vi "Echo.vi"(4 "Magnitude":dbl=0.5, 6 "Delay ms:":i32=5000, 7 "Input":path) -> (5 "output":path)   [LabVIEW 2012]
panel:
  out "Waveform Graph 2":waveform(dbl)(graph)
  out "Waveform Graph":waveform(dbl)(graph)
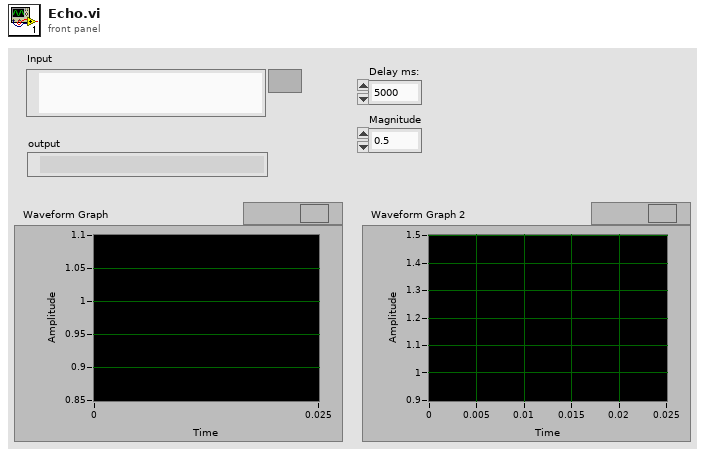
[diagram p1: front panel]
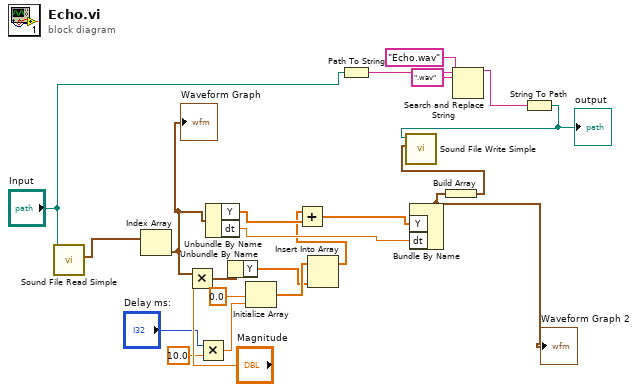
[diagram p0: block diagram]
diagram:
  n1 = call <vilib>:"Sound File Read Simple.vi"("path"="Input") -> ("data"=w22:waveform(dbl)[])  [unwired: 7 in, 3 out]
  n2 = Index Array(array=w22) -> (element=w18:waveform(dbl))  [unwired: 1 in]
  "Waveform Graph" <- w18
  n3 = Multiply(x=w18, y="Magnitude") -> (x*y=w15:waveform(dbl))
  n4 = Multiply(x="Delay ms:", y=10.0) -> (x*y=w11:dbl)
  n5 = Unbundle By Name(w18) -> ("Y"=w8:dbl[], "dt"=w17:dbl)
  n6 = Unbundle By Name(w15) -> ("Y"=w14:dbl[])
  n7 = Initialize Array(0.0 ("element"), w11) -> (w19:dbl[])
  n8 = Insert Into Array(array=w19, new element=w14) -> (w7:dbl[])  [unwired: 1 in]
  n9 = Add(x=w7, y=w8) -> (x+y=w13:dbl[])
  n10 = Path To String(path="Input") -> (string=w5:string)
  n11 = Bundle By Name("Y"=w13, "dt"=w17) -> (w12:waveform(dbl))  [unwired: 1 in]
  "Waveform Graph 2" <- w12
  n12 = Build Array(w12) -> (w16:waveform(dbl)[])
  n13 = Search and Replace String(input string=w5, search string=".wav", replace string="Echo.wav" ("replace string (\"\")")) -> (result string=w2:string)  [unwired: 5 in, 3 out]
  n14 = String To Path(string=w2) -> (path=w1:path)
  "output" <- w1
  n15 = call <vilib>:"Sound File Write Simple.vi"("data"=w16, "path"=w1) -> ()  [unwired: 8 in, 2 out]
